vi "SMC MagStatus= Message.vi"(0 "Sweep Status":enum16{"Hold", "To Setpoint", "To Zero"}(ring)) -> ()   [LabVIEW 2010]
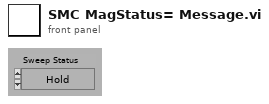
[diagram p1: front panel]
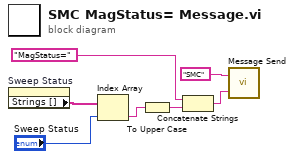
[diagram p0: block diagram]
diagram:
  n1 = property on="Sweep Status" class="Enum (strict)"() -> ("Strings []"=w3:string[])  [unwired: 2 in, 2 out]
  n2 = Index Array(array=w3, index="Sweep Status") -> (element=w1:string)
  n3 = To Upper Case(1:w1) -> (0:w4:string)
  n4 = Concatenate Strings("MagStatus=" ("Message"), w4) -> (w7:string)
  n5 = call "Message Send.vi"("Message"=w7, "Destination"="SMC" ("Destination(s)")) -> ()
